vi "Harmonikgerilim_Tablo_Doldur.vi"(10 "Table Reference in":refnum<vi>) -> (1 "Test Result":bool, 2 "Table Values":string[][](array[string]))   [LabVIEW 2014]
uses:
  TestStandInteraction/VeriPaylasim_Globali.vi
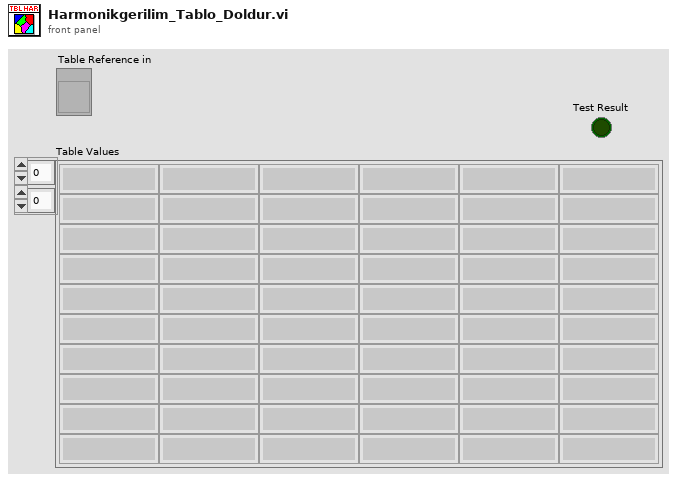
[diagram p1: front panel]
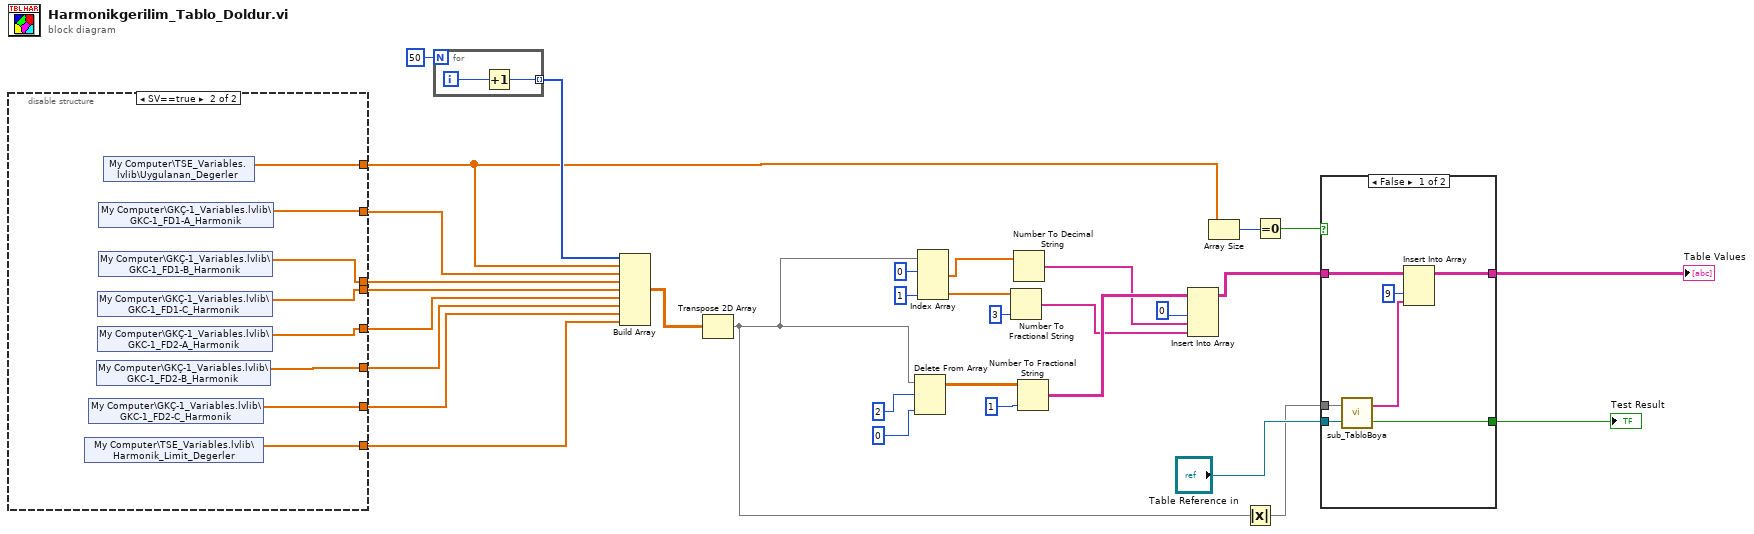
[diagram p0: block diagram]
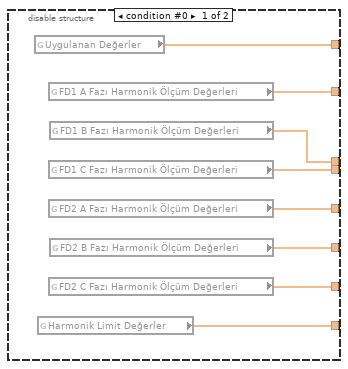
[diagram p2: hidden frame]
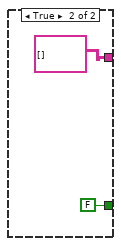
[diagram p3: hidden frame]
diagram:
  n1 = disable-structure shown="SV==true" {
    disable-tunnel: [w40 w48] -> w1
    disable-tunnel: [w39 w46] -> w9
    disable-tunnel: [w38 w45] -> w8
    disable-tunnel: [w37 w44] -> w7
    disable-tunnel: [w36 w43] -> w6
    disable-tunnel: [w35 w42] -> w5
    disable-tunnel: [w34 w41] -> w4
    disable-tunnel: [w33 w47] -> w3
    frame condition #0 {
      n2 = global read "VeriPaylasim_Globali.vi" "Uygulanan Değerler"() -> (w40:dbl[])
      n3 = global read "VeriPaylasim_Globali.vi" "Harmonik Limit Değerler"() -> (w33:dbl[])
      n4 = global read "VeriPaylasim_Globali.vi" "FD1 A Fazı Harmonik Ölçüm Değerleri"() -> (w39:dbl[])
      n5 = global read "VeriPaylasim_Globali.vi" "FD1 C Fazı Harmonik Ölçüm Değerleri"() -> (w37:dbl[])
      n6 = global read "VeriPaylasim_Globali.vi" "FD2 A Fazı Harmonik Ölçüm Değerleri"() -> (w36:dbl[])
      n7 = global read "VeriPaylasim_Globali.vi" "FD2 C Fazı Harmonik Ölçüm Değerleri"() -> (w34:dbl[])
      n8 = global read "VeriPaylasim_Globali.vi" "FD1 B Fazı Harmonik Ölçüm Değerleri"() -> (w38:dbl[])
      n9 = global read "VeriPaylasim_Globali.vi" "FD2 B Fazı Harmonik Ölçüm Değerleri"() -> (w35:dbl[])
    }
    frame condition #1 (active) {
      n10 = shared-variable "My Computer\\TSE_Variables.lvlib\\Harmonik_Limit_Degerler"() -> (w47:dbl[])  [unwired: 1 in, 1 out]
      n11 = shared-variable "My Computer\\GKÇ-1_Variables.lvlib\\GKC-1_FD2-C_Harmonik"() -> (w41:dbl[])  [unwired: 1 in, 1 out]
      n12 = shared-variable "My Computer\\GKÇ-1_Variables.lvlib\\GKC-1_FD2-B_Harmonik"() -> (w42:dbl[])  [unwired: 1 in, 1 out]
      n13 = shared-variable "My Computer\\GKÇ-1_Variables.lvlib\\GKC-1_FD1-C_Harmonik"() -> (w44:dbl[])  [unwired: 1 in, 1 out]
      n14 = shared-variable "My Computer\\GKÇ-1_Variables.lvlib\\GKC-1_FD2-A_Harmonik"() -> (w43:dbl[])  [unwired: 1 in, 1 out]
      n15 = shared-variable "My Computer\\GKÇ-1_Variables.lvlib\\GKC-1_FD1-A_Harmonik"() -> (w46:dbl[])  [unwired: 1 in, 1 out]
      n16 = shared-variable "My Computer\\GKÇ-1_Variables.lvlib\\GKC-1_FD1-B_Harmonik"() -> (w45:dbl[])  [unwired: 1 in, 1 out]
      n17 = shared-variable "My Computer\\TSE_Variables.lvlib\\Uygulanan_Degerler"() -> (w48:dbl[])  [unwired: 1 in, 1 out]
    }
  }
  n18 = for {
    N: 50 -> [_]
    tunnel: [w49] -> w10 mode=indexing
    i -> [w50]
    n19 = Increment(x=w50) -> (x+1=w49:i32)
  }
  n20 = Build Array(w10, w1, w9, w8, w7, w6, w5, w4, w3) -> (w2:dbl[][])
  n21 = Transpose 2D Array(2D array=w2) -> (transposed array=w21:dbl[][])
  n22 = Delete From Array "Delete From Array"(array=w21, length=2, index (col)=0 ("disabled index (col)")) -> (array with subset deleted=w23:dbl[][])  [unwired: 1 in, 1 out]
  n23 = Index Array "Index Array"(array=w21, index (col) #1=0 ("disabled index (col)"), index (col) #2=1 ("disabled index (col)")) -> (element #1=w18:dbl[], element #2=w25:dbl[])  [unwired: 2 in]
  n24 = Number To Fractional String(number=w25, precision (6)=i16 3) -> (F-format string=w15:string[])  [unwired: 2 in]
  n25 = Number To Decimal String(number=w18) -> (decimal integer string=w16:string[])  [unwired: 1 in]
  n26 = Number To Fractional String(number=w23, precision (6)=i16 1) -> (F-format string=w17:string[][])  [unwired: 2 in]
  n27 = Insert Into Array(array=w17, index (col)=0 ("disabled index (col)"), new element #1=w16, new element #2=w15) -> (w13:string[][])  [unwired: 1 in]
  n28 = Array Size(array=w1) -> (size(s)=w30:i32)
  n29 = Absolute Value(x=w21) -> (abs(x)=w12:dbl[][])
  n30 = Equal To 0?(x=w30) -> (x = 0?=w29:bool)
  n31 = case shown="False" w29 {
    tunnel: "Table Reference in" -> [w57 _]
    tunnel: w12 -> [w56 _]
    tunnel: w13 -> [w55 _]
    tunnel: [w52 FALSE ("Test Result")] -> w31
    tunnel: [w51 string[][] []] -> w28
    frame False {
      n32 = call "sub_TabloBoya.vi"("Table in"=w57, "Tablo Degerleri"=w56) -> ("Test Result"=w52:bool, "RESULTS"=w54:string[])
      n33 = Insert Into Array(array=w55, index (col)=9 ("disabled index (col)"), new element=w54) -> (w51:string[][])  [unwired: 1 in]
    }
    frame True {
    }
  }
  "Table Values" <- w28
  "Test Result" <- w31
